vi "Gyro.vi"   [LabVIEW 2016, in "FPGAMockGyro.lvlib"]
uses:
  FPGAMockGyro.lvlib
  FPGA/ModbusCRC32Settings.ctl
  <vilib>/Platform/TimedLoop/XDataNode/timing_clust.ctl
  <vilib>/Platform/TimedLoop/XDataNode/nitl_modes.ctl
  <vilib>/Platform/TimedLoop/XDataNode/wakeup.ctl
  DataTypes/GyroData.ctl
  DataTypes/GyroStates.ctl
  <vilib>/rvi/Emulation/niFpgaGetClockAttributes.vi
  <vilib>/rvi/Emulation/niFpgaSctlEmulationGetInTimedLoop.vi
  <vilib>/rvi/Emulation/niFpgaEmulationReportErrorSimple.vi
  <vilib>/rvi/interface/RandomDataEmulation/niFpgaRandomDataHandleErrors.vi
  <vilib>/rvi/Memory/Memory_Emulation/nirvimemoryFastEmulation.vi
  <vilib>/rvi/Memory/Memory_Emulation/nirvimemoryEmulation.vi
  <vilib>/rvi/Emulation/niFpgaEmulationIsFPGAContextNoSignature.vi
  <vilib>/rvi/DataTransferAndStorage/Container/Common/niFpgaContainerGetUniqueNameForEmu.vi
  <vilib>/rvi/Emulation/niFpgaProcessEmulError.vi
  <vilib>/rvi/errors/nirviReportUnexpectedCaseInternalError (U32).vi
  <vilib>/rvi/Emulation/niFpgaCriticalErrorInLSC.vi
  <vilib>/rvi/errors/niFpgaSetErrorForExecOnDevCompSimple.vi
  <vilib>/rvi/eio/common/nirviEmuReportErrorAndStop.vi
  <vilib>/rvi/FIFO/Fifo_Resource/nirvififoEmulationSetSize.vi
  <vilib>/rvi/FIFO/Fifo_Resource/nirviFifoEmulationQueueMgr.vi
  <instcachedir>/0/nirviFifoEmulationQueueMgr_E5CAEC123FF24DC58D834DCA3CDAA9B5.lvgen/nirviFifoEmulationQueueMgr_E5CAEC123FF24DC58D834DCA3CDAA9B5_009.vi
  <vilib>/Utility/error.llb/Clear Errors.vi
  <vilib>/rvi/FIFO/Fifo_Resource/nirvififoEmulationCreateLock.vi
  <vilib>/rvi/FIFO/Fifo_Resource/nirvififoEmulationObtainLock.vi
  <vilib>/rvi/FIFO/Fifo_Resource/nirvififoEmulationReleaseLock.vi
  <vilib>/rvi/occurrence/nirviWaitOnOccurrenceBase.vi
  <vilib>/rvi/errors/nirviReportUnexpectedCaseInternalError.vi
  <instcachedir>/0/nirviFifoEmulationQueueMgr_E5CAEC123FF24DC58D834DCA3CDAA9B5.lvgen/nirviFifoEmulationQueueMgr_E5CAEC123FF24DC58D834DCA3CDAA9B5_002.vi
  <vilib>/rvi/FIFO/Fifo_Resource/nirvififoEmulationDetermineInputValidOut.vi
  <instcachedir>/0/nirviFifoEmulationQueueMgr_E5CAEC123FF24DC58D834DCA3CDAA9B5.lvgen/nirviFifoEmulationQueueMgr_E5CAEC123FF24DC58D834DCA3CDAA9B5_004.vi
  <vilib>/rvi/DataTransferAndStorage/Container/XNode/niFpgaContainer.xnode
  <vilib>/rvi/interface/RandomDataEmulation/nirviRandomDataFpgaReadWriteTemplate.vi
  <vilib>/Platform/TimedLoop/XDataNode/XDataNode.xnode
  <vilib>/rvi/FIFO/Fifo_Resource/nirvififoEmulationRead.vi
  <vilib>/rvi/FIFO/Fifo_Resource/nirvififoEmulationWrite.vi
  <vilib>/Platform/TimedLoop/XDataNode/XDNodeRunTimeDep.lvlib
types:
  T1 = typedef "ModbusCRC32Settings.ctl" = cluster{"DataFIFO":refnum<k21>, "CalculateFIFO":refnum<k21>, "OutputFIFO":refnum<k21>}
  T2 = typedef "FPGAMockGyro.lvlib/GyroData.ctl" = cluster{"GyroStates":T3, "Index":u32}
  T3 = typedef "FPGAMockGyro.lvlib/GyroStates.ctl" = enum8{"TxData", "TxCRC", "Delay"}
  T4 = typedef "XDNodeRunTimeDep.lvlib/timing_clust.ctl" = cluster{"Expected End [f-1]":u64, "Actual End [f-1]":u64, "Finished Late? [f-1]":bool, "Expected End [i-1]":u64, "Actual End [i-1]":u64, "Finished Late? [i-1]":bool, "Expected Start [i]":u64, "Actual Start [i]":u64, "Expected Start [f]":u64, "Actual Start [f]":u64, "Source Name":string, "Structure Name":string, "Period":i64, "Deadline":i64, "Offset":i64, "Start":i64, "Priority":i32, "Timeout":i32, "Mode":T5, "Wakeup Reason":T6, "Error":errorcluster, "Source Type":string, "Secondary Source Type":string, "Global End Time":u64, "Global Start Time":u64, "Frame Duration":u64, "Iteration Duration":u64, "Assigned CPU":i32, "I/O Scan Engine Mode":u32}
  T5 = typedef "XDNodeRunTimeDep.lvlib/nitl_modes.ctl" = enum32{"No Change", "Process missed periods, maintain original phase", "Discard missed periods, maintain original phase", "Process missed periods, ignore original phase", "Discard missed periods, ignore original phase"}
  T6 = typedef "XDNodeRunTimeDep.lvlib/wakeup.ctl" = enum32{"Normal", "Aborted", "Asynchronous wakeup", "Timing source error", "Timed loop error", "Timeout"}
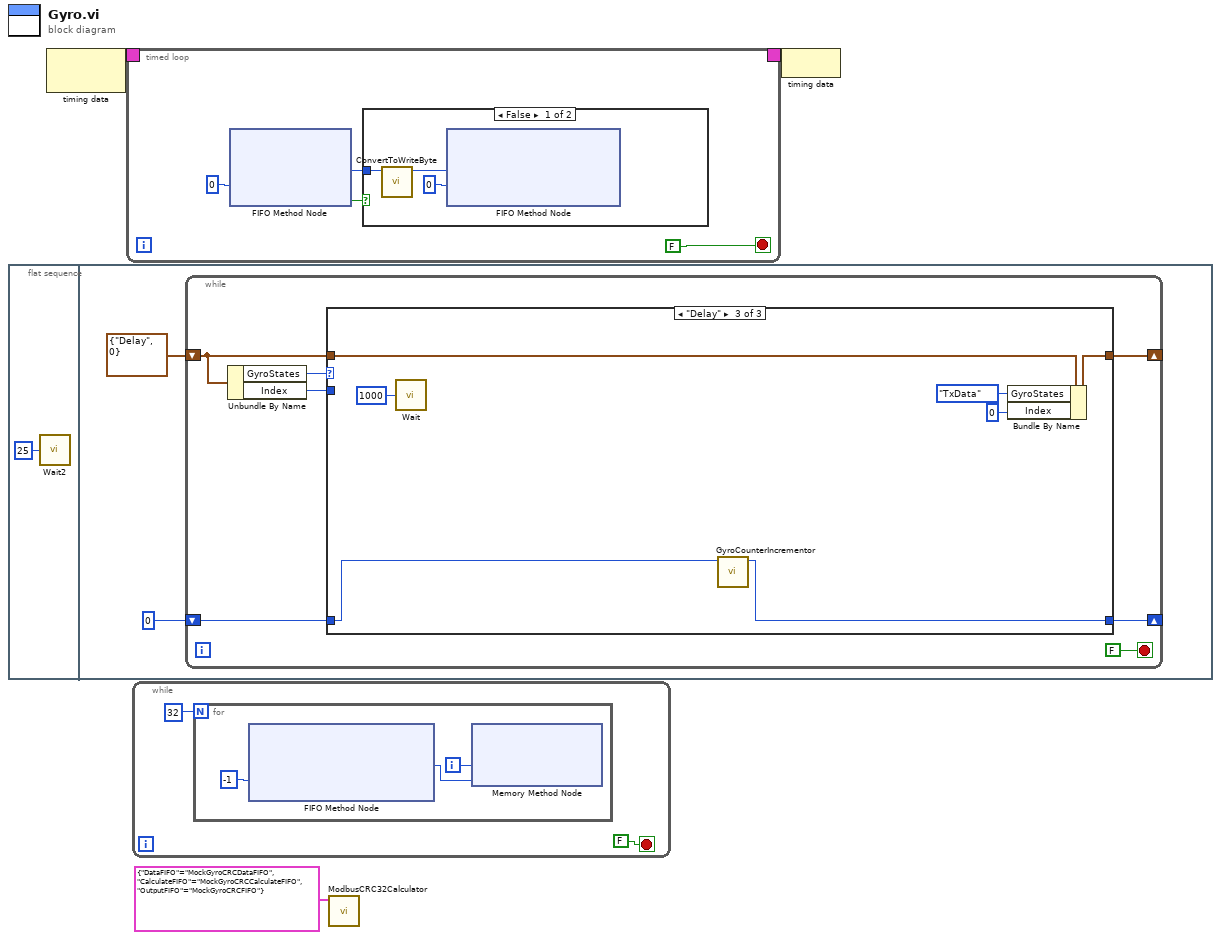
[diagram p0: block diagram]
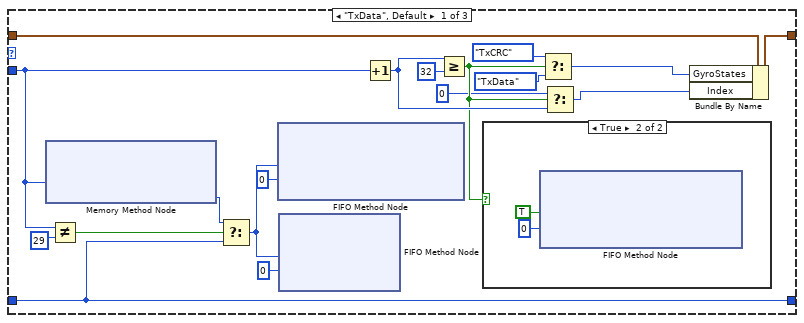
[diagram p2: hidden frame]
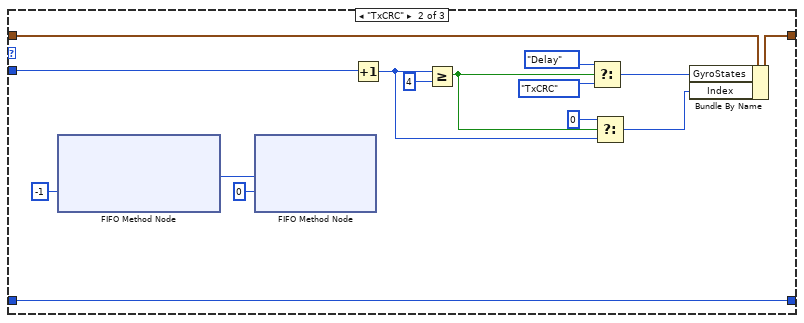
[diagram p4: hidden frame]
diagram:
  n1 = flat-sequence {
    frame #0 {
      n2 = call "Wait2"("Count(mSec)"=u32 25) -> ()  [unwired: 1 out]
    }
    frame #1 {
      n3 = while {
        shift-right: [w11] -> _
        shift-left: T2 {"GyroStates"=enum."Delay", "Index"=0} ("GyroData") -> [w10]
        shift-right: [w7] -> _
        shift-left: u8 0 -> [w8]
        stop <- FALSE stop-if-true
        n4 = Unbundle By Name(w10) -> ("GyroStates"=w13:T3, "Index"=w12:u32)
        n5 = case shown="\"Delay\"" w13 {
          tunnel: w12 -> [w23 w42 _]
          tunnel: [w24 w47 w54] -> w11
          tunnel: w10 -> [w25 w48 w55]
          tunnel: w8 -> [w18 w43 w51]
          tunnel: [w18 w43 w50] -> w7
          frame "TxData", Default {
            n6 = xnode ("Memory Method Node")("Address"=w23) -> ("Data"=w21:u8)  [unwired: 1 in, 1 out]
            n7 = Not Equal?(x=w23, y=u32 29) -> (x != y?=w20:bool)
            n8 = Select(t=w21, s=w20, f=w18) -> (s? t:f=w19:u8)
            n9 = xnode ("FIFO Method Node")("Element"=w19, "Timeout"=0) -> ()  [unwired: 1 in, 2 out]
            n10 = xnode ("FIFO Method Node")("Element"=w19, "Timeout"=0) -> ()  [unwired: 1 in, 2 out]
            n11 = Increment(x=w23) -> (x+1=w17:u32)
            n12 = Greater Or Equal?(x=w17, y=u32 32) -> (x >= y?=w16:bool)
            n13 = case shown="True" w16 {
              frame False {
              }
              frame True {
                n14 = xnode ("FIFO Method Node")("Element"=TRUE, "Timeout"=0) -> ()  [unwired: 1 in, 2 out]
              }
            }
            n15 = Select(t=GyroStates."TxCRC", s=w16, f=GyroStates."TxData" ("GyroStates")) -> (s? t:f=w26:T3)
            n16 = Select(t=u32 0, s=w16, f=w17) -> (s? t:f=w14:u32)
            n17 = Bundle By Name(cluster=w25, "GyroStates"=w26, "Index"=w14) -> (w24:T2)
          }
          frame "TxCRC" {
            n18 = xnode ("FIFO Method Node")("Timeout"=-1) -> ("Element"=w45:u8)  [unwired: 1 in, 2 out]
            n19 = xnode ("FIFO Method Node")("Element"=w45, "Timeout"=0) -> ()  [unwired: 1 in, 2 out]
            n20 = Increment(x=w42) -> (x+1=w37:u32)
            n21 = Greater Or Equal?(x=w37, y=u32 4) -> (x >= y?=w36:bool)
            n22 = Select(t=GyroStates."Delay" ("GyroStates"), s=w36, f=GyroStates."TxCRC") -> (s? t:f=w38:T3)
            n23 = Select(t=u32 0, s=w36, f=w37) -> (s? t:f=w34:u32)
            n24 = Bundle By Name(cluster=w48, "GyroStates"=w38, "Index"=w34) -> (w47:T2)
          }
          frame "Delay" {
            n25 = call "Wait"("Count(uSec)"=u32 1000 ("Count(mSec)")) -> ()  [unwired: 1 out]
            n26 = call "GyroCounterIncrementor.vi"("CurrentCounter"=w51) -> ("NewCounter"=w50:u8)  [unwired: 10 in]
            n27 = Bundle By Name(cluster=w55, "GyroStates"=GyroStates."TxData", "Index"=u32 0) -> (w54:T2)
          }
        }
      }
    }
  }
  n28 = node-c288() -> (w3:T4)  [unwired: 1 in]
  n29 = timed-loop {
    timing: w3 -> [_]
    timing-out: [_] -> w2
    stop <- FALSE stop-if-true
    n30 = xnode ("FIFO Method Node")("Timeout"=0) -> ("Element"=w57:u8, "Timed Out?"=w58:bool)  [unwired: 1 in, 1 out]
    n31 = case shown="False" w58 {
      tunnel: w57 -> [w62 _]
      frame False {
        n32 = call "ConvertToWriteByte.vi"("Input"=w62) -> ("Output"=w61:u16)  [unwired: 10 in]
        n33 = xnode ("FIFO Method Node")("Element"=w61, "Timeout"=0) -> ()  [unwired: 1 in, 2 out]
      }
      frame True {
      }
    }
  }
  n34 = while {
    stop <- FALSE stop-if-true
    n35 = for {
      N: 32 -> [_]
      i -> [w68]
      n36 = xnode ("FIFO Method Node")("Timeout"=-1) -> ("Element"=w67:u8)  [unwired: 1 in, 2 out]
      n37 = xnode ("Memory Method Node")("Address"=w68, "Data"=w67) -> ()  [unwired: 1 in, 1 out]
    }
  }
  n38 = call "ModbusCRC32Calculator.vi"("ModbusCRC32Settings"=T1 {"DataFIFO"="MockGyroCRCDataFIFO", "CalculateFIFO"="MockGyroCRCCalculateFIFO", "OutputFIFO"="MockGyroCRCFIFO"}) -> ()  [unwired: 11 in]
  n39 = node-c288(w2) -> ()
